vi "Read ADC Measurement Process.vi"(7 "Measurement Started?":bool, 8 "error in (no error)":errorcluster, 11 "Session Handle in":T1) -> (0 "error out":errorcluster, 2 "Passed?":bool, 3 "Session Handle out":T1 caption="Gas")   [LabVIEW 2015]
uses:
  Typedefs/Session Handle.ctl
  PAS.lvclass
panel:
  out "Frequency":dbl
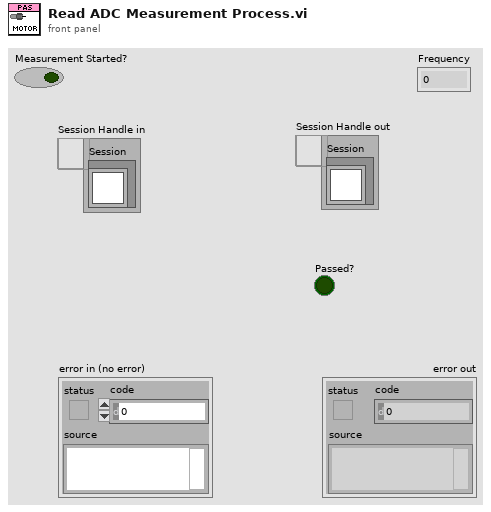
[diagram p1: front panel]
types:
  T1 = typedef "PAS.lvclass/Session Handle.ctl" = refnum<data-value>
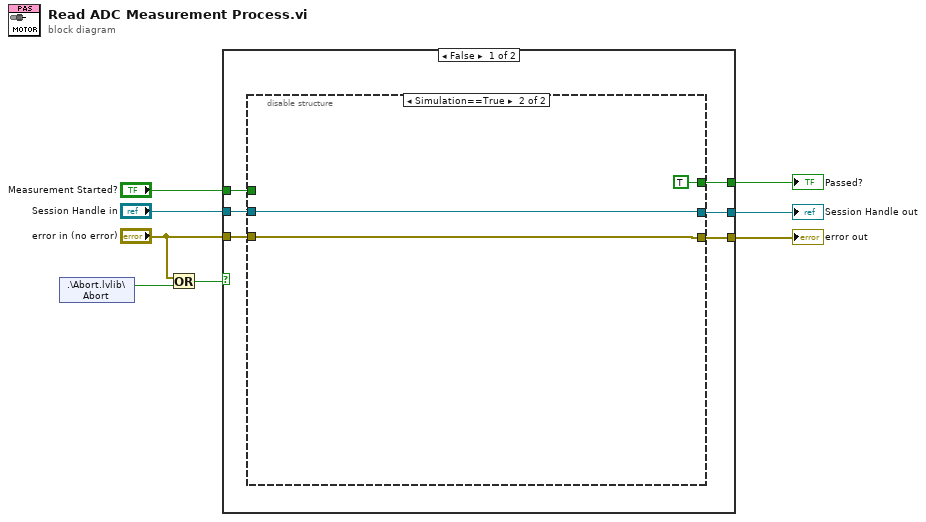
[diagram p0: block diagram]
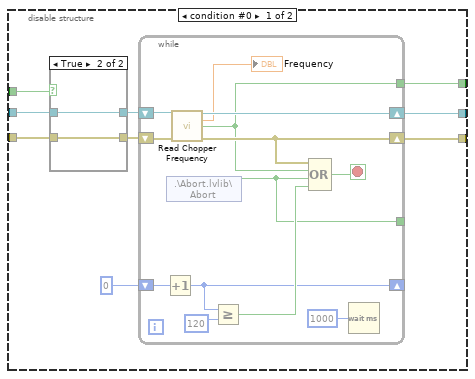
[diagram p2: hidden frame]
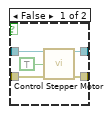
[diagram p3: hidden frame]
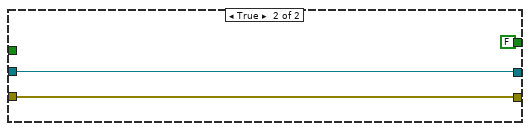
[diagram p4: hidden frame]
diagram:
  n1 = shared-variable ".\\Abort.lvlib\\Abort"() -> (w3:bool)  [unwired: 1 in, 1 out]
  n2 = Or(x="error in (no error)", y=w3) -> (x .or. y?=w2:bool)
  n3 = case shown="False" w2 {
    tunnel: [w9 w47] -> w8
    tunnel: "Session Handle in" -> [w14 w48]
    tunnel: "error in (no error)" -> [w13 w47]
    tunnel: [w10 FALSE ("Finished Ramping?")] -> w6
    tunnel: [w11 w48] -> w5
    tunnel: "Measurement Started?" -> [w12 _]
    frame False {
      n4 = disable-structure shown="Simulation==True" {
        disable-tunnel: w14 -> [w21 w46]
        disable-tunnel: w13 -> [w20 w45]
        disable-tunnel: w12 -> [w18 _]
        disable-tunnel: [w17 w46] -> w11
        disable-tunnel: [w16 TRUE ("Finished Ramping?")] -> w10
        disable-tunnel: [w15 w45] -> w9
        frame condition #0 {
          n5 = case shown="True" w18 {
            tunnel: [w28 w30] -> w23
            tunnel: [w27 w29] -> w22
            tunnel: w21 -> [w26 w30]
            tunnel: w20 -> [w25 w29]
            frame False {
              n6 = call "Control Stepper Motor.vi"("Session Handle in"=w26, "Start?"=TRUE, "error in (no error)"=w25) -> ("Session Handle out"=w28:T1, "error out"=w27:errorcluster)  [unwired: 10 in, 1 out]
            }
            frame True {
            }
          }
          n7 = while {
            shift-right: [w39] -> w15
            shift-left: w22 -> [w42]
            shift-right: [w41] -> w17
            shift-left: w23 -> [w43]
            tunnel: [w37] -> w16
            shift-right: [w33] -> _
            shift-left: u32 0 ("milliseconds to wait") -> [w36]
            tunnel: [w31] -> _
            stop <- w38 stop-if-true
            n8 = Increment(x=w36) -> (x+1=w33:u32)
            n9 = shared-variable ".\\Abort.lvlib\\Abort"() -> (w31:bool)  [unwired: 1 in, 1 out]
            n10 = call "Read Chopper Frequency.vi"("Session Handle in"=w43, "error in (no error)"=w42) -> ("Session Handle out"=w41:T1, "Frequency"=→"Frequency":dbl, "Finished Ramping?"=w37:bool, "error out"=w39:errorcluster)  [unwired: 9 in, 1 out]
            n11 = Greater Or Equal?(x=w33, y=u32 120) -> (x >= y?=w34:bool)
            n12 = Compound Arithmetic op=OR(w39, w37, w31, w34) -> (w38:bool)
            n13 = Wait (ms)(milliseconds to wait=u32 1000) -> ()  [unwired: 1 out]
          }
        }
        frame condition #1 (active) {
        }
      }
    }
    frame True {
    }
  }
  "error out" <- w8
  "Passed?" <- w6
  "Session Handle out" <- w5
